vi "test_arduino.vi"() -> ()   [LabVIEW 2018]
uses:
  <vilib>/Instr/_visa.llb/VISA Configure Serial Port (Instr).vi
panel:
  in  "VISA resource name":refnum<visa-resource-name>="COM9"
  in  "Read (0, default)/Write (1)":bool
  in  "State":bool
  in  "Pin Num":u32=2 min=2 max=12
  out "Bytes at Port":u32
  out "read buffer":string
  # "click this"
  # "so, maybe you can do it yourself, just run this and see\nwhat you see on the scope"
  # "0: all ok\n3: state requested was not 0/1\nother: ???"
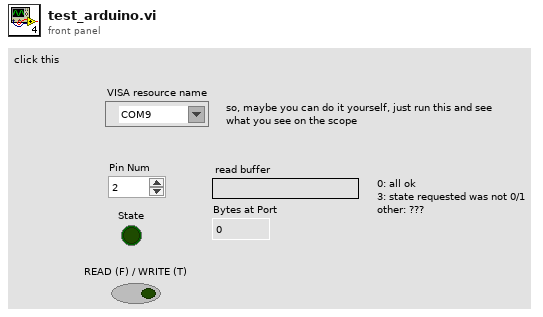
[diagram p1: front panel]
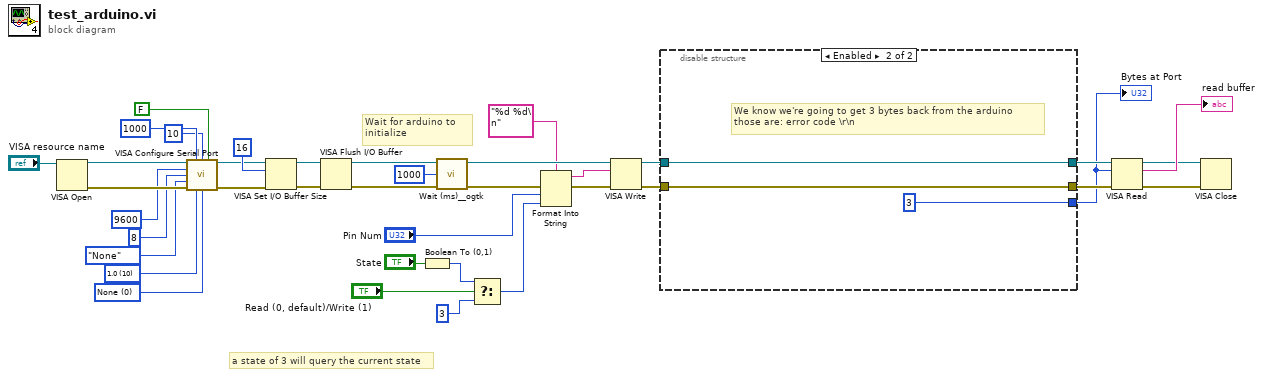
[diagram p0: block diagram]
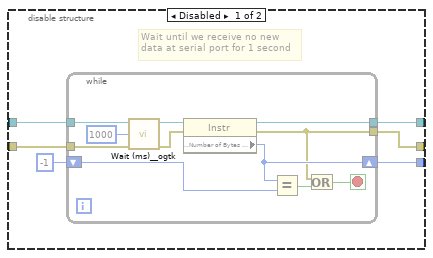
[diagram p2: hidden frame]
diagram:
  w30 = u16 0 items=["None", "XON/XOFF", "RTS/CTS", "XON/XOFF & RTS/CTS", "DTR/DSR", "XON/XOFF & DTR/DSR"] ("flow control (0:none)")
  w31 = u16 10 items=["1.0"=10, "1.5"=15, "2.0"=20] ("stop bits (10: 1 bit)")
  # "a state of 3 will query the current state"
  # "Wait for arduino to\ninitialize"
  n1 = VISA Open(VISA resource name="VISA resource name") -> (VISA resource name=w37:refnum<visa-resource-name>, error out=w36:errorcluster)  [unwired: 4 in]
  n2 = call-poly "VISA Configure Serial Port"("VISA resource name"=w37, "timeout (10sec)"=u32 1000, "termination char\n(0xA = '\\n' = LF)"=u8 10 ("termination char\n(0xA = '\\n' = LF)"), "Enable Termination\nChar (T)"=FALSE ("Enable Termination\nChar (T)"), "baud rate (9600)"=u32 9600, "data bits (8)"=u16 8, "parity (0:none)"=enum16{"None", "Odd", "Even", "Mark", "Space"}."None", "error in (no error)"=w36, "stop bits (10: 1 bit)"=w31, "flow control (0:none)"=w30) -> ("VISA resource name out"=w15:refnum<visa-resource-name>, "error out"=w14:errorcluster)  [unwired: 4 in]
  n3 = VISA Set I/O Buffer Size(VISA resource name=w15, mask (16)=u16 16 ("I/O Receive\nBuffer mask"), error in (no error)=w14) -> (VISA resource name out=w16:refnum<visa-resource-name>, error out=w13:errorcluster)  [unwired: 1 in]
  n4 = VISA Flush I/O Buffer(VISA resource name=w16, error in (no error)=w13) -> (VISA resource name out=w28:refnum<visa-resource-name>, error out=w10:errorcluster)  [unwired: 1 in]
  n5 = Boolean To (0,1)(Boolean="State") -> (0, 1=w5:i16)
  n6 = call <userlib>:"Wait (ms)__ogtk.vi"("error in (no error)"=w10, "milliseconds to wait"=u32 1000) -> ("error out"=w9:errorcluster)  [unwired: 8 in, 1 out]
  n7 = Select(t=w5, s="Read (0, default)/Write (1)", f=i16 3 ("t")) -> (s? t:f=w4:i16)
  n8 = Format Into String(format string="%d %d\n", error in=w9, "Pin Num", w4) -> (resulting string=w2:string, error out=w29:errorcluster)  [unwired: 1 in]
  n9 = VISA Write(VISA resource name=w28, write buffer=w2, error in (no error)=w29) -> (VISA resource name out=w24:refnum<visa-resource-name>, error out=w23:errorcluster)  [unwired: 1 out]
  n10 = disable-structure shown="Enabled" {
    disable-tunnel: w24 -> [w43 w55]
    disable-tunnel: w23 -> [w42 w56]
    disable-tunnel: [w40 w55] -> w22
    disable-tunnel: [w39 w56] -> w21
    disable-tunnel: [w38 u32 3 ("Bytes at Port")] -> w18
    frame Disabled {
      # "Wait until we receive no new \ndata at serial port for 1 second"
      n11 = while {
        tunnel: w43 -> [w53]
        tunnel: w42 -> [w50]
        shift-right: [w48] -> w38
        shift-left: -1 ("timeout (10sec)") -> [w49]
        tunnel: [w47] -> w40
        tunnel: [w44] -> w39
        stop <- w46 stop-if-true
        n12 = call <userlib>:"Wait (ms)__ogtk.vi"("error in (no error)"=w50, "milliseconds to wait"=u32 1000) -> ("error out"=w51:errorcluster)  [unwired: 8 in, 1 out]
        n13 = property class="Instr"(reference=w53, error in=w51) -> (reference out=w47:refnum<visa-resource-name>, error out=w44:errorcluster, "Serial Settings:Number of Bytes at Serial Port"=w48:u32)
        n14 = Equal?(x=w48, y=w49) -> (x = y?=w45:bool)
        n15 = Or(x=w44, y=w45) -> (x .or. y?=w46:bool)
      }
    }
    frame Enabled {
      # "We know we're going to get 3 bytes back from the arduino\nthose are: error code \\r\\n"
    }
  }
  "Bytes at Port" <- w18
  n16 = VISA Read(VISA resource name=w22, byte count=w18, error in (no error)=w21) -> (VISA resource name out=w1:refnum<visa-resource-name>, read buffer=→"read buffer":string, error out=w20:errorcluster)  [unwired: 1 out]
  n17 = VISA Close(VISA resource name=w1, error in (no error)=w20) -> ()  [unwired: 1 out]
